vi "ATF-Pump-Check loop Error_R.vi"(4 "Ignore Errors":i32[](array[numeric]), 6 "Log-Only Errors":i32[](array[numeric]), 9 "Critical Errors":i32[](array[numeric]), 10 "error to process":errorcluster, 11 "Message Queue":refnum<queue>) -> (2 "Enqueued Error?":bool, 3 "dup Message Queue":refnum<queue>)   [LabVIEW 2022 SP3]
uses:
  RT Controls/Message Cluster_R.ctl
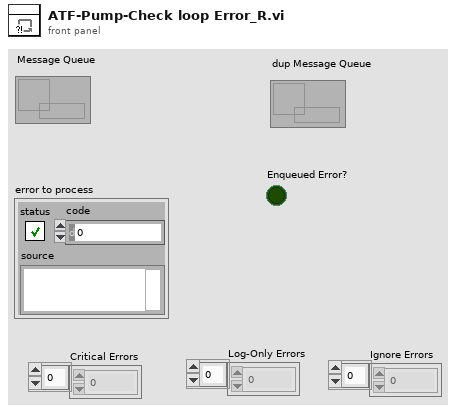
[diagram p1: front panel]
types:
  T1 = enum16{"Log-Only Error", "Non-Critical Error", "Critical Error"}
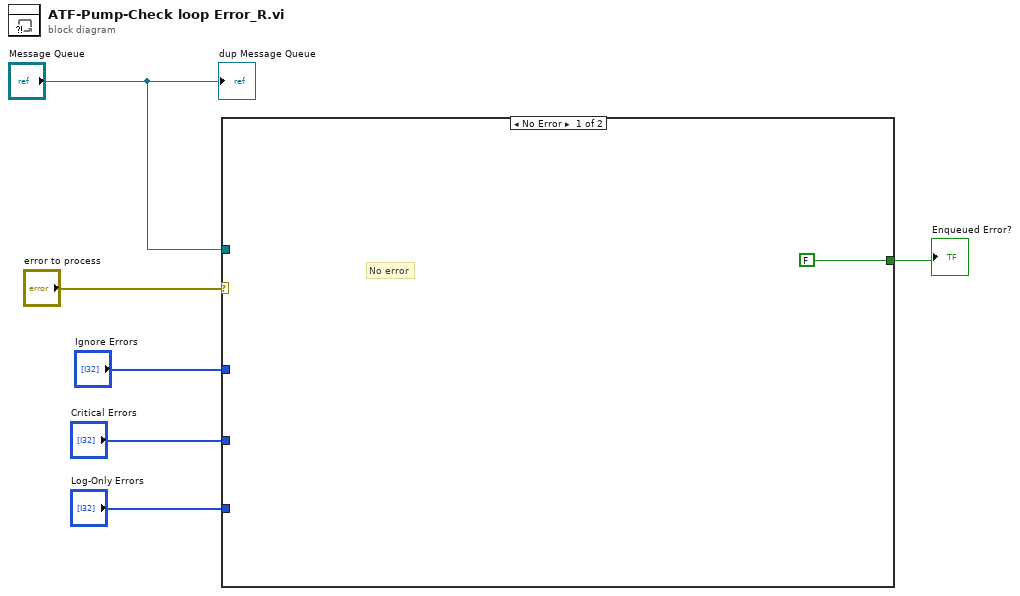
[diagram p0: block diagram]
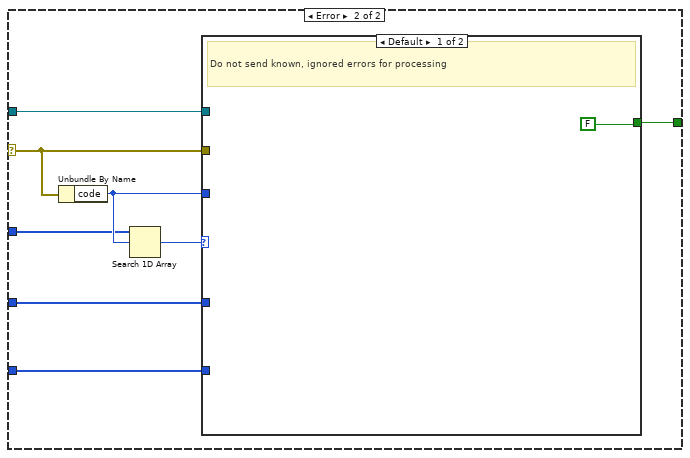
[diagram p2: hidden frame]
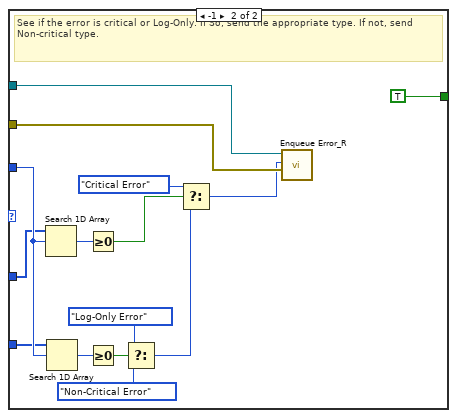
[diagram p3: hidden frame]
diagram:
  n1 = case shown="No Error" "error to process" {
    selector: "error to process" -> [_ w14]
    tunnel: "Message Queue" -> [_ w15]
    tunnel: "Ignore Errors" -> [_ w11]
    tunnel: "Critical Errors" -> [_ w10]
    tunnel: "Log-Only Errors" -> [_ w9]
    tunnel: [FALSE w8] -> w1
    frame No Error {
      # "No error"
    }
    frame Error {
      n2 = Unbundle By Name(w14) -> ("code"=w13:i32)
      n3 = Search 1D Array(1D array=w11, element=w13) -> (index of element=w12:i32)  [unwired: 1 in]
      n4 = case shown="Default" w12 {
        tunnel: w14 -> [_ w31]
        tunnel: w15 -> [_ w30]
        tunnel: w13 -> [_ w20]
        tunnel: w10 -> [_ w19]
        tunnel: w9 -> [_ w18]
        tunnel: [FALSE TRUE] -> w8
        frame Default {
          # "Do not send known, ignored errors for processing"
        }
        frame -1 {
          # "See if the error is critical or Log-Only. If So, send the appropriate type. If not, send Non-critical type."
          n5 = Search 1D Array(1D array=w19, element=w20) -> (index of element=w22:i32)  [unwired: 1 in]
          n6 = Search 1D Array(1D array=w18, element=w20) -> (index of element=w23:i32)  [unwired: 1 in]
          n7 = Greater Or Equal To 0?(x=w22) -> (x >= 0?=w24:bool)
          n8 = Greater Or Equal To 0?(x=w23) -> (x >= 0?=w26:bool)
          n9 = Select(t=T1."Log-Only Error" ("Error Type (Non-Critical)"), s=w26, f=T1."Non-Critical Error" ("Error Type (Non-Critical)")) -> (s? t:f=w28:T1)
          n10 = Select(t=T1."Critical Error" ("Error Type (Non-Critical)"), s=w24, f=w28) -> (s? t:f=w21:T1)
          n11 = call "Enqueue Error_R.vi"("error to process"=w31, "Error Type (Non-Critical)"=w21, "Message Queue"=w30) -> ()  [unwired: 9 in]
        }
      }
    }
  }
  "Enqueued Error?" <- w1
  "dup Message Queue" <- "Message Queue"
